vi "MagMountSelect.vi"(9 "Mounted Chip(G)":enum32{"1", "2", "3", "4", "5", "6", "7", "8"}[](array[ring])=[enum."1", enum."2", enum."3", enum."4"], 11 "Calibrated B(G)":dbl[][](array[numeric])=[[-0.3967537201699907, 0.339914475525817, -2.21781660383778], [-0.3017004124305834, 0.280101884974311, -1.6794955825651372], [-0.41686059975821277, -0.2595882338977341, -1.6329741725277818], [-0.29750658257693735, -0.18769541419704472, -1.013820871986511]]) -> (3 "Mounted Chip(G)":dbl[][](array[numeric]))   [LabVIEW 2012]
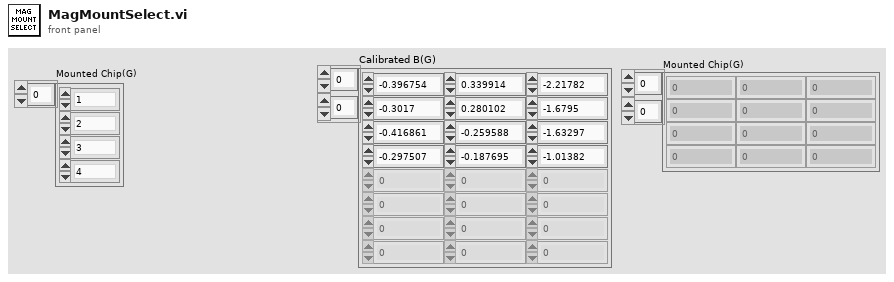
[diagram p1: front panel]
types:
  T1 = cluster{"Mounted Chip(G)[0]":enum32{"1", "2", "3", "4", "5", "6", "7", "8"}, "Mounted Chip(G)[1]":enum32{"1", "2", "3", "4", "5", "6", "7", "8"}, "Mounted Chip(G)[2]":enum32{"1", "2", "3", "4", "5", "6", "7", "8"}, "Mounted Chip(G)[3]":enum32{"1", "2", "3", "4", "5", "6", "7", "8"}, "Mounted Chip(G)[4]":enum32{"1", "2", "3", "4", "5", "6", "7", "8"}, "Mounted Chip(G)[5]":enum32{"1", "2", "3", "4", "5", "6", "7", "8"}, "Mounted Chip(G)[6]":enum32{"1", "2", "3", "4", "5", "6", "7", "8"}, "Mounted Chip(G)[7]":enum32{"1", "2", "3", "4", "5", "6", "7", "8"}, "Mounted Chip(G)[8]":enum32{"1", "2", "3", "4", "5", "6", "7", "8"}}
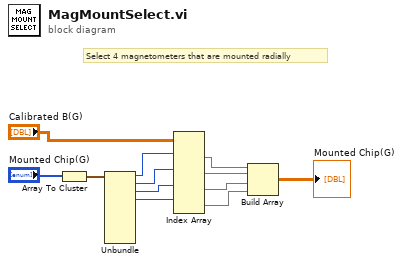
[diagram p0: block diagram]
diagram:
  # "Select 4 magnetometers that are mounted radially"
  n1 = Array To Cluster(array="Mounted Chip(G)") -> (cluster=w10:T1)
  n2 = Unbundle(w10) -> ("Mounted Chip(G)[0]"=w9:enum32{"1", "2", "3", "4", "5", "6", "7", "8"}, "Mounted Chip(G)[1]"=w8:enum32{"1", "2", "3", "4", "5", "6", "7", "8"}, "Mounted Chip(G)[2]"=w7:enum32{"1", "2", "3", "4", "5", "6", "7", "8"}, "Mounted Chip(G)[3]"=w6:enum32{"1", "2", "3", "4", "5", "6", "7", "8"})  [unwired: 5 out]
  n3 = Index Array(array="Calibrated B(G)", index (row) #1=w9, index (row) #2=w8, index (row) #3=w7, index (row) #4=w6) -> (element #1=w5:dbl[], element #2=w4:dbl[], element #3=w3:dbl[], element #4=w2:dbl[])  [unwired: 4 in]
  n4 = Build Array(w5, w4, w3, w2) -> (→"Mounted Chip(G)":dbl[][])
